vi "GT Get Auto Focus Status.vi"(8 "error in (no error)":errorcluster caption="错误输入（无错误）", 9 "count":i16, 10 "pStatus":u16, 11 "cardNum":i16) -> (0 "error out":errorcluster caption="错误输出", 2 "pStatus out":u16, 3 "function return":i16)   [LabVIEW 2014, in "gts.lvlib"]
doc: "GT_API GT_GetAutoFocusStatus(short cardNum,unsigned short *pStatus,short count);"
uses:
  gts.lvlib
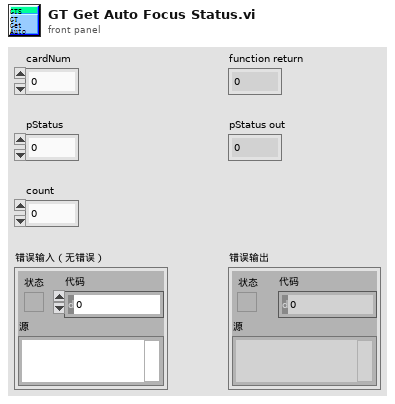
[diagram p1: front panel]
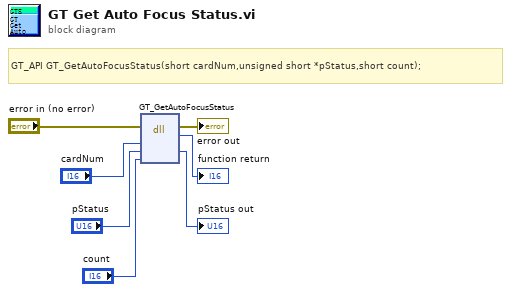
[diagram p0: block diagram]
diagram:
  # "GT_API GT_GetAutoFocusStatus(short cardNum,unsigned short *pStatus,short count);"
  n1 = dll-call lib="PTH2habs D固高科技资料GTS控制卡GTS卡18年上半年资料dllVC32bit\nmulti_cardgts.*" fn="GT_GetAutoFocusStatus"(error in="error in (no error)", "cardNum"="cardNum", "pStatus"="pStatus", "count"="count") -> (error out=→"error out":errorcluster, →"function return":i16, "pStatus"=→"pStatus out":u16)  [unwired: 4 in, 1 out]
